vi "Find RT Systems.vi"(8 "error in (no error)":errorcluster, 9 "Cancel In Reference":refnum<vi>, 10 "Progress Reference In":refnum<vi>, 11 "Timeout ms (4000)":i32=4000) -> (0 "error out":errorcluster, 1 "Progress Reference Out":refnum<vi>, 2 "Cancel Out":refnum<vi>, 3 "All RT Info":T1(array[cluster]))   [LabVIEW 2015]
uses:
  <vilib>/nisyscfg/nisyscfg.lvlib
  <resource>/objmgr/nisysapi.rc
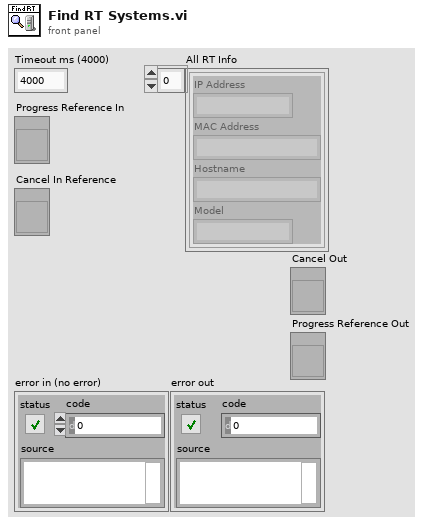
[diagram p1: front panel]
types:
  T1 = cluster{"IP Address":string, "MAC Address":string, "Hostname":string, "Model":string}[]
  T2 = cluster{"IP Address":string, "MAC Address":string, "Hostname":string, "Model":string}
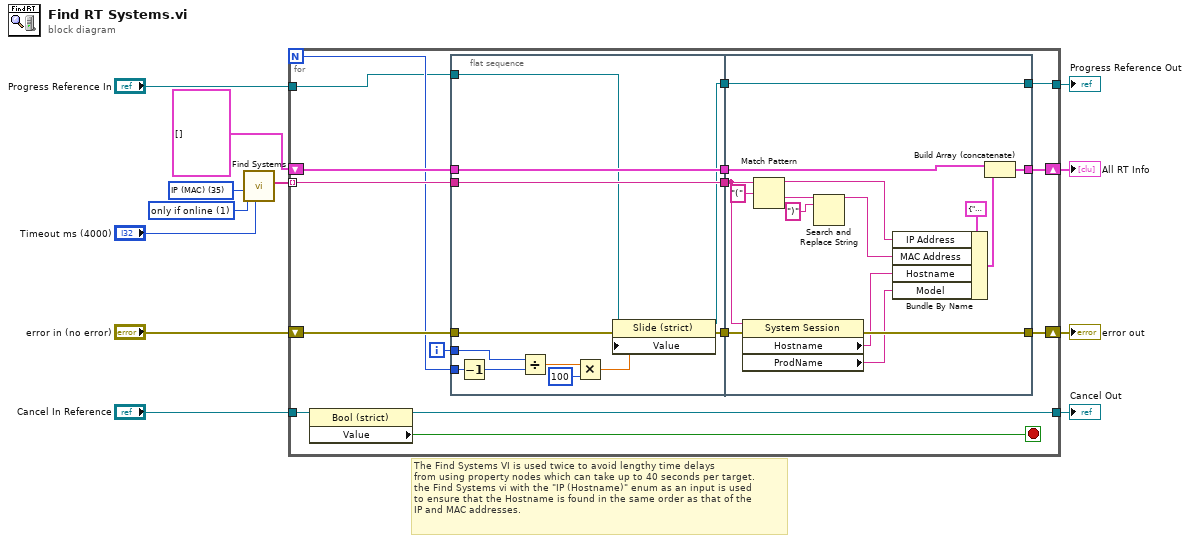
[diagram p0: block diagram]
diagram:
  w4 = u32 1 items=["none"=0, "only if online"=1, "all"=3] ("Include Cached Results (all)")
  w12 = u32 35 items=["Hostname"=16, "Hostname (IP)"=18, "Hostname (MAC)"=19, "IP"=32, "IP (Hostname)"=33, "IP (MAC)"=35, "MAC"=48, "MAC (Hostname)"=49, "MAC (IP)"=50] ("Output (Hostname and IP)")
  # "The Find Systems VI is used twice to avoid lengthy time delays\nfrom using property nodes which can take up to 40 seconds per target.\nthe Find Systems vi with the \"IP (Hostname)\" enum as an input is used\nto ensure that the Hostname is found in the same order as that of the \nIP and MAC addresses."
  n1 = call <vilib>:"Find Systems.vi"("Timeout (4000 ms)"="Timeout ms (4000)", "Output (Hostname and IP)"=w12, "Include Cached Results (all)"=w4) -> ("Detected Systems"=w11:string[])  [unwired: 6 in, 2 out]
  n2 = for {
    N -> [w19]
    tunnel: w11 -> [w28] mode=indexing
    shift-right: [w27] -> w9
    shift-left: T1 [] -> [w26]
    shift-right: [w24] -> w7
    shift-left: "error in (no error)" -> [w25]
    tunnel: "Progress Reference In" -> [w16]
    tunnel: [w18] -> w1
    tunnel: "Cancel In Reference" -> [w15]
    tunnel: [w13] -> w2
    i -> [w20]
    stop <- w14 stop-if-true
    n3 = property class="Bool (strict)"(reference=w15) -> (reference out=w13:refnum<vi>, "Value"=w14:bool)  [unwired: 1 in, 1 out]
    n4 = flat-sequence {
      tunnel: w25 -> [w30]
      tunnel: w26 -> [w39]
      tunnel: w28 -> [w40]
      tunnel: [w40] -> w23
      tunnel: [w39] -> w22
      tunnel: [w29] -> w21
      tunnel: w20 -> [w34]
      tunnel: w19 -> [w33]
      tunnel: [w32] -> w17
      tunnel: w16 -> [w31]
      tunnel: [w48] -> w27
      tunnel: [w45] -> w24
      tunnel: w23 -> [w43]
      tunnel: w22 -> [w47]
      tunnel: w21 -> [w46]
      tunnel: [w44] -> w18
      tunnel: w17 -> [w44]
      frame #0 {
        n5 = Decrement(x=w33) -> (x-1=w36:i32)
        n6 = Divide(x=w34, y=w36) -> (x/y=w37:dbl)
        n7 = Multiply(x=w37, y=u32 100) -> (x*y=w38:dbl)
        n8 = property class="Slide (strict)"(reference=w31, error in=w30, "Value"=w38) -> (reference out=w32:refnum<vi>, error out=w29:errorcluster)
      }
      frame #1 {
        n9 = property class="System Session"(reference=w43, error in=w46) -> (error out=w45:errorcluster, "Hostname"=w42:string, "ProdName"=w41:string)  [unwired: 1 out]
        n10 = Match Pattern(string=w43, regular expression="(") -> (before substring=w50:string, after substring=w54:string)  [unwired: 1 in, 2 out]
        n11 = Search and Replace String(input string=w54, search string=")") -> (result string=w49:string)  [unwired: 6 in, 3 out]
        n12 = Bundle By Name(cluster=T2 {"IP Address"="", "MAC Address"="", "Hostname"="", "Model"=""} ("input cluster"), "IP Address"=w50, "MAC Address"=w49, "Hostname"=w42, "Model"=w41) -> (w52:T2)
        n13 = Build Array (concatenate)(w47, w52) -> (w48:T1)
      }
    }
  }
  "All RT Info" <- w9
  "error out" <- w7
  "Cancel Out" <- w2
  "Progress Reference Out" <- w1
